vi "Set Temperature and Wait.vi"(0 "Comms Port":refnum<visa-resource-name>="COM1", 1 "Accuracy +/-":dbl=0.25 format="%.3g", 11 "Error In":errorcluster, 12 "Set Point":dbl=33.0 format="%.3g", 13 "Seconds":i32, 14 "close session(t)":bool=TRUE) -> (6 "ILabVIEW":refnum<k24>, 15 "error out":errorcluster)   [LabVIEW 2018]
uses:
  C:/RageATE/Instruments/Ess Temp Plate/LabView Driver/Public/Watbus.dll
  LabView Driver/Public/Watbus.dll
panel:
  out "Waveform Chart 2":dbl(graph)=31.97
  out "Temp 2":dbl=31.97
  out "Set Point (str)":string="33.000"
  in  "Refresh Rate(s)":dbl=1.0 format="%#_13g"
  in  "Stop":bool=TRUE
  out "Temp":dbl=31.97
  out "LSL":dbl=32.75
  out "USL":dbl=33.25
  in  "deviceType":i32(ring) items=["Controller", "RUI", "PC", "CommsCard"]
  in  "InstanceId":i32=1
  in  "Zone":i32=1
  in  "RO(t)":bool
  in  "TemperatureUnits":u8(ring)=1 items=["Degrees F", "Degrees C"]
  out "Waveform Chart":dbl(graph)=31.97
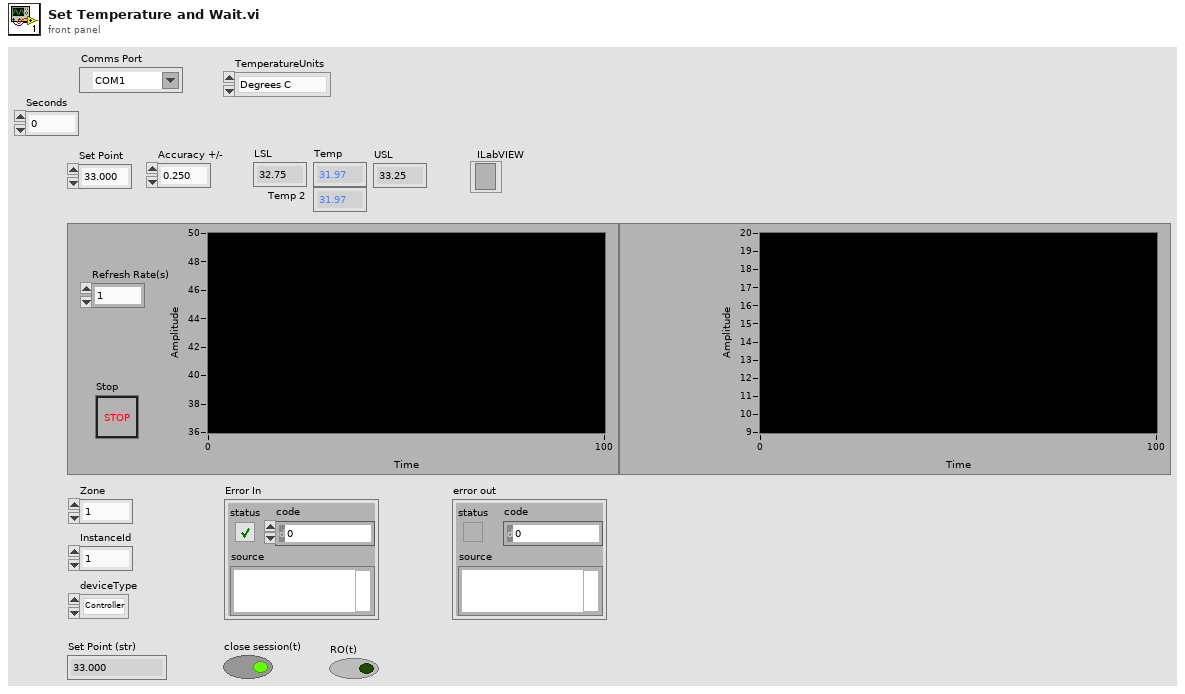
[diagram p1: front panel]
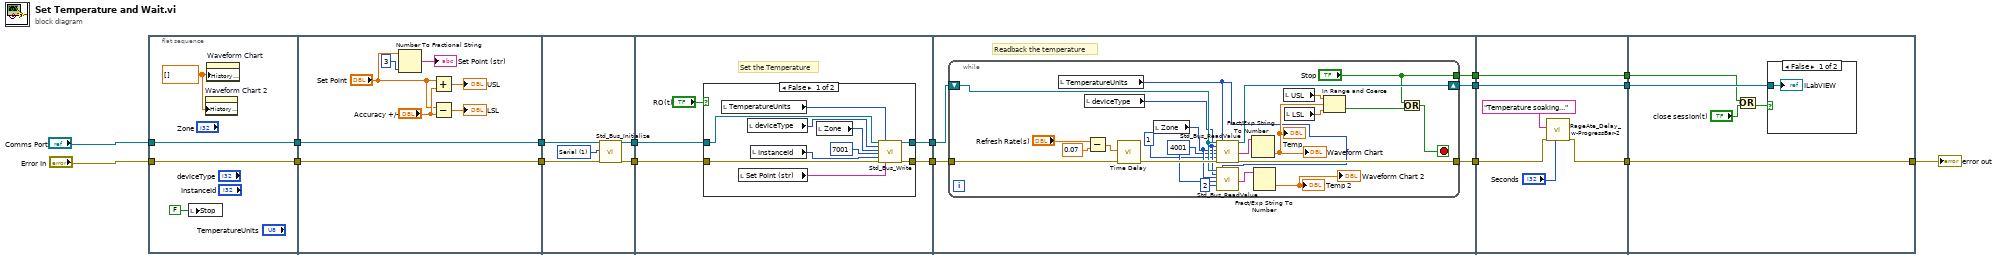
[diagram p0: block diagram]
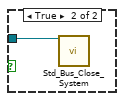
[diagram p3: hidden frame]
diagram:
  n1 = flat-sequence {
    tunnel: "Error In" -> [w20]
    tunnel: "Comms Port" -> [w21]
    tunnel: [w21] -> w9
    tunnel: [w20] -> w8
    tunnel: [w29] -> w11
    tunnel: [w28] -> w10
    tunnel: w9 -> [w29]
    tunnel: w8 -> [w28]
    tunnel: [w30] -> w15
    tunnel: [w31] -> w14
    tunnel: w11 -> [w34]
    tunnel: w10 -> [w32]
    tunnel: [w36] -> w17
    tunnel: [w35] -> w16
    tunnel: w15 -> [w38]
    tunnel: w14 -> [w37]
    tunnel: [w54] -> w6
    tunnel: [w53] -> w4
    tunnel: w17 -> [w56]
    tunnel: w16 -> [w55]
    tunnel: [w52] -> w2
    tunnel: w6 -> [w85]
    tunnel: [w85] -> w5
    tunnel: w4 -> [w81]
    tunnel: [w80] -> w3
    tunnel: w2 -> [w84]
    tunnel: [w84] -> w1
    tunnel: w5 -> [w90]
    tunnel: w3 -> [w89]
    tunnel: [w89] -> w7
    tunnel: w1 -> [w86]
    frame #0 {
      w18 = dbl[] [] ("History Data")
      n2 = local write "Stop"(FALSE ("Stop")) -> ()
      n3 = property on="Waveform Chart 2" class="WFChart (strict)"("History Data"=w18) -> ()  [unwired: 2 in, 2 out]
      n4 = property on="Waveform Chart" class="WFChart (strict)"("History Data"=w18) -> ()  [unwired: 2 in, 2 out]
    }
    frame #1 {
      n5 = Number To Fractional String(number="Set Point", precision (6)=i16 3) -> (F-format string=→"Set Point (str)":string)  [unwired: 2 in]
      n6 = Add(x="Set Point", y="Accuracy +/-") -> (x+y=→"USL":dbl)
      n7 = Subtract(x="Set Point", y="Accuracy +/-") -> (x-y=→"LSL":dbl)
    }
    frame #2 {
      w33 = 1 items=["Usb", "Serial", "Ethernet", "Unconnected"] ("InterfaceType")
      n8 = call "Std_Bus_Initialize.vi"("Communications Port"=w34, "InterfaceType"=w33, "error in (no error)"=w32) -> ("ILabVIEW"=w31:refnum<k24>, "error out"=w30:errorcluster)  [unwired: 14 in, 1 out]
    }
    frame #3 {
      # "Set the Temperature"
      n9 = case shown="False" "RO(t)" {
        tunnel: [w49 w50] -> w36
        tunnel: [w48 w51] -> w35
        tunnel: w38 -> [w47 w51]
        tunnel: w37 -> [w46 w50]
        frame False {
          n10 = local read "TemperatureUnits"() -> (w40:u8)
          n11 = local read "Set Point (str)"() -> (w41:string)
          n12 = local read "deviceType"() -> (w43:i32)
          n13 = local read "InstanceId"() -> (w42:i32)
          n14 = local read "Zone"() -> (w44:i32)
          n15 = call "Std_Bus_Write.vi"("ILabVIEW In"=w46, "deviceType"=w43, "Zone"=w44, "ParameterID"=7001, "InstanceId"=w42, "error in (no error)"=w47, "TemperatureUnits"=w40, "WriteValue"=w41) -> ("ILabVIEW Out"=w49:refnum<k24>, "error out"=w48:errorcluster)  [unwired: 10 in]
        }
        frame True {
        }
      }
    }
    frame #4 {
      # "Readback the temperature"
      n16 = while {
        tunnel: w55 -> [w79]
        shift-right: [w78] -> w54
        shift-left: w56 -> [w65]
        tunnel: [w68] -> w53
        tunnel: ["Stop"] -> w52
        stop <- w72 stop-if-true
        w62 = 4001 ("ParameterID")
        n17 = local read "TemperatureUnits"() -> (w58:u8)
        n18 = local read "deviceType"() -> (w64:i32)
        n19 = Subtract(x="Refresh Rate(s)", y=0.07) -> (x-y=w70:dbl)
        n20 = call "Time Delay"("error in (no error)"=w79, "Delay Time (s)"=w70) -> ("error out"=w77:errorcluster)  [unwired: 9 in]
        n21 = local read "Zone"() -> (w63:i32)
        n22 = call "Std_Bus_ReadValue.vi"("ILabVIEW In"=w65, "DeviceType"=w64, "Zone"=w63, "ParameterID"=w62, "InstanceId"=1, "error in (no error)"=w77, "TemperatureUnits"=w58) -> ("ILabVIEW Out"=w78:refnum<k24>, "Value Out"=w76:string, "error out"=w68:errorcluster)  [unwired: 10 in]
        n23 = call "Std_Bus_ReadValue.vi"("ILabVIEW In"=w65, "DeviceType"=w64, "Zone"=w63, "ParameterID"=w62, "InstanceId"=2, "TemperatureUnits"=w58) -> ("Value Out"=w59:string)  [unwired: 11 in, 2 out]
        n24 = Fract/Exp String To Number(string=w76) -> (number=w67:dbl)  [unwired: 3 in, 1 out]
        "Temp" <- w67
        "Waveform Chart" <- w67
        n25 = Fract/Exp String To Number(string=w59) -> (number=→"Temp 2" →"Waveform Chart 2":dbl)  [unwired: 3 in, 1 out]
        n26 = local read "USL"() -> (w75:dbl)
        n27 = local read "LSL"() -> (w74:dbl)
        n28 = In Range and Coerce(upper limit=w75, x=w67, lower limit=w74) -> (In Range?=w73:bool)  [unwired: 1 out]
        n29 = Or(x="Stop", y=w73) -> (x .or. y?=w72:bool)
      }
    }
    frame #5 {
      n30 = call "RageAte_Delay_w-ProgressBar-2.vi"("Seconds"="Seconds", "error in (no error)"=w81, "Delay text ..."="Temperature soaking...") -> ("error out"=w80:errorcluster)  [unwired: 8 in]
    }
    frame #6 {
      n31 = Or(x=w86, y="close session(t)") -> (x .or. y?=w87:bool)
      n32 = case shown="False" w87 {
        tunnel: w90 -> [w91 w92]
        frame False {
          "ILabVIEW" <- w91
        }
        frame True {
          n33 = call "Std_Bus_Close_System.vi"("ILabVIEW In"=w92) -> ()  [unwired: 18 in, 1 out]
        }
      }
    }
  }
  "error out" <- w7
